vi "Init.vi"(8 "error in (no error)":errorcluster, 11 "uService Template in":refnum<class "Kasli Listener.lvclass">) -> (0 "error out":errorcluster, 3 "uService Template out":refnum<class "Kasli Listener.lvclass">)   [LabVIEW 2020, in "CIRCUS_uServices.lvlib" / "Kasli Listener and Writer.lvlib" / "Kasli Listener.lvclass"]
uses:
  Kasli Listener.lvclass
  LabVIEW/builds/TALOS/TALOS_PPL.lvlibp/Internal uServices/System uServices/TCP Listener/TCP Listener/TCP Listener.lvclass
  LabVIEW/builds/TALOS/TALOS_PPL.lvlibp/Ancestor/Ancestor/Ancestor.lvclass
  LabVIEW/builds/TALOS/TALOS_PPL.lvlibp/Father of all uServices/Father of all uServices/Father of all uServices.lvclass
  C:/LabVIEW/builds/TALOS/TALOS_PPL.lvlibp/Ancestor/Ancestor/Ancestor.lvclass
  C:/LabVIEW/builds/TALOS/TALOS_PPL.lvlibp/Father of all uServices/Father of all uServices/Father of all uServices.lvclass
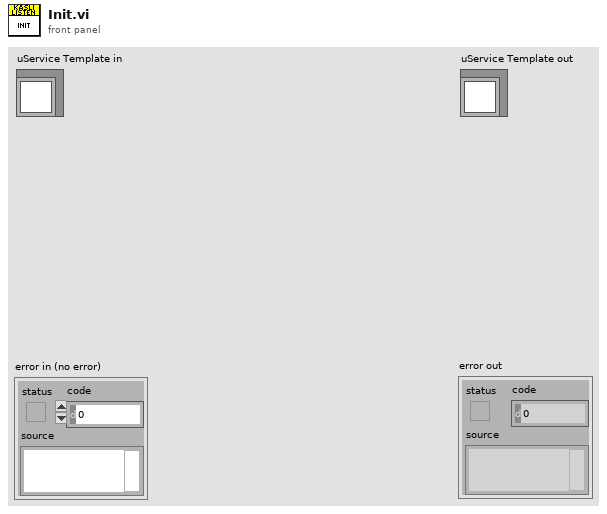
[diagram p1: front panel]
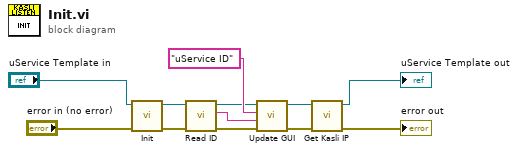
[diagram p0: block diagram]
diagram:
  n1 = call-parent "Init.vi"("error in (no error)"="error in (no error)", "uService Template in"="uService Template in") -> ("error out"=w3:errorcluster, "uService Template out"=w6:refnum<class "Kasli Listener.lvclass">)  [unwired: 8 in]
  n2 = call "Read ID.vi"("error in (no error)"=w3, "Ancestor in"=w6) -> ("error out"=w2:errorcluster, "ID"=w8:string, "Ancestor out"=w5:refnum<class "Kasli Listener.lvclass">)  [unwired: 7 in]
  n3 = call "Update GUI.vi"("error in (no error)"=w2, "Data"=w8, "GUI Item Name"="uService ID", "uService Template in"=w5) -> ("error out"=w1:errorcluster, "uService Template out"=w4:refnum<class "Kasli Listener.lvclass">)  [unwired: 6 in]
  n4 = call-dynamic "Get Kasli IP.vi"("error in (no error)"=w1, "Kasli Listener in"=w4) -> ("error out"=→"error out":errorcluster, "Kasli Listener out"=→"uService Template out":refnum<class "Kasli Listener.lvclass">)  [unwired: 8 in]
